vi "Gateway_Reply.vi"(8 "error in (no error)":errorcluster, 11 "GatewayClass in":refnum<class "GatewayClass.lvclass">) -> (0 "error out":errorcluster, 2 "JSON Bytes sent":i32, 3 "GatewayClass out":refnum<class "GatewayClass.lvclass">)   [LabVIEW 2018, in "GatewayClass.lvclass"]
uses:
  GatewayClass.lvclass
  GatewayClass.lvclass/GatewayClass.ctl
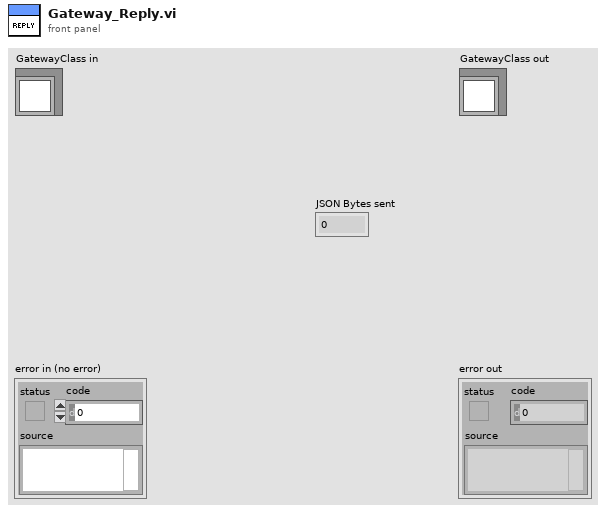
[diagram p1: front panel]
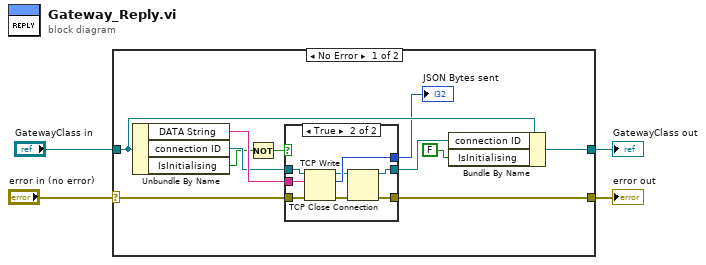
[diagram p0: block diagram]
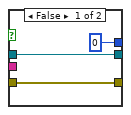
[diagram p2: hidden frame]
diagram:
  n1 = case shown="No Error" "error in (no error)" {
    selector: "error in (no error)" -> [w15 w28]
    tunnel: [w12 w28] -> w3
    tunnel: [w8 w27] -> w1
    tunnel: "GatewayClass in" -> [w11 w27]
    frame No Error {
      n2 = Unbundle By Name(w11) -> ("DATA String"=w14:string, "connection ID"=w13:refnum<k5>, "IsInitialising"=w7:bool)
      n3 = Not(x=w7) -> (.not. x?=w6:bool)
      n4 = case shown="True" w6 {
        tunnel: w15 -> [w17 w26]
        tunnel: w13 -> [w18 w25]
        tunnel: [w17 w20] -> w12
        tunnel: [0 ("bytes written") w24] -> w9
        tunnel: [w18 w22] -> w10
        tunnel: w14 -> [_ w19]
        frame False {
        }
        frame True {
          n5 = TCP Write(connection ID=w25, data in=w19, error in (no error)=w26) -> (connection ID out=w23:refnum<k5>, bytes written=w24:i32, error out=w21:errorcluster)  [unwired: 1 in]
          n6 = TCP Close Connection(connection ID=w23, error in (no error)=w21) -> (connection ID out=w22:refnum<k5>, error out=w20:errorcluster)  [unwired: 1 in]
        }
      }
      "JSON Bytes sent" <- w9
      n7 = Bundle By Name(cluster=w11, "connection ID"=w10, "IsInitialising"=FALSE) -> (w8:refnum<class "GatewayClass.lvclass">)
    }
    frame Error {
    }
  }
  "error out" <- w3
  "GatewayClass out" <- w1
